vi "test_examples.vi"(9 "expectations":cluster{"label":string, "<JSON>value":string}[](array[cluster]), 10 "controls":cluster{"label":string, "<JSON>value":string}[](array[cluster]), 11 "file":string) -> (0 "error out":errorcluster)   [LabVIEW 2017, in "example_tests.lvlib"]
uses:
  example_tests.lvlib
  de0021a5-3447-4bd8-a116-6765a7690623.vi
  f64fb9af-96c6-48b4-92cc-20c95939fb08.vi
  libssh2/libssh2_init_default.vi
  <vilib>/JDP Science/JSONtext/JSON text to Variant.vi
  <vilib>/JDP Science/JSONtext/Variant to JSON Text.vi
  <vilib>/JDP Science/JSONtext/LVClass Serializer/JSONtext LVClass Serializer.lvclass
  libssh2/libssh2.lvlib
  <vilib>/JDP Science/JSONtext/JSONtext.lvlib
  <vilib>/PNR/Transparent Assertions/Transparent Assertions/Transparent Assertions.lvlib
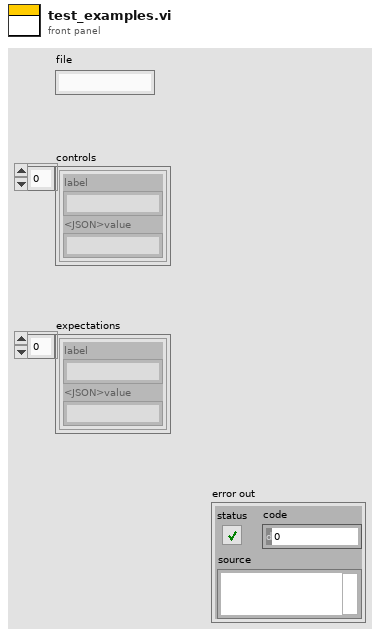
[diagram p1: front panel]
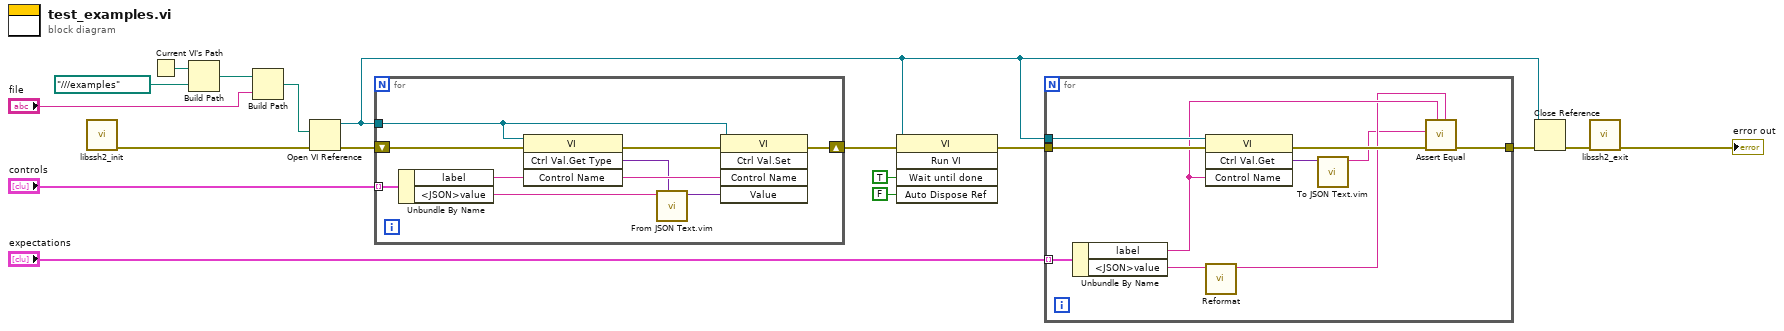
[diagram p0: block diagram]
diagram:
  n1 = call-poly "libssh2_init.vi"() -> ("error out"=w15:errorcluster)  [unwired: 11 in]
  n2 = Current VI's Path() -> (path=w11:path)
  n3 = Build Path(base path=w11, name or relative path=path "../../../examples" ("path")) -> (appended path=w9:path)
  n4 = Build Path(base path=w9, name or relative path="file") -> (appended path=w8:path)
  n5 = Open VI Reference(vi path=w8, error in (no error)=w15) -> (vi reference=w6:refnum<vi>, error out=w13:errorcluster)  [unwired: 4 in]
  n6 = for {
    tunnel: "controls" -> [w26] mode=indexing
    shift-right: [w25] -> w12
    shift-left: w13 -> [w23]
    tunnel: w6 -> [w24]
    n7 = Unbundle By Name(w26) -> ("label"=w22:string, "<JSON>value"=w20:string)
    n8 = invoke on="Invoke Node" class="VI" method="Ctrl Val.Get Type"(reference=w24, error in=w23, "Control Name"=w22) -> (error out=w18:errorcluster, "Ctrl Val.Get Type"=w21:variant)  [unwired: 1 in, 2 out]
    n9 = call "From JSON Text.vim"("Data Type and Default Value"=w21, "JSON"=w20) -> ("Data out"=w19:variant)  [unwired: 8 in, 1 out]
    n10 = invoke on="Invoke Node" class="VI" method="Ctrl Val.Set"(reference=w24, error in=w18, "Control Name"=w22, "Value"=w19) -> (error out=w25:errorcluster)  [unwired: 1 in, 4 out]
  }
  n11 = invoke on="Invoke Node" class="VI" method="Run VI"(reference=w6, error in=w12, "Wait until done"=TRUE ("Wait Until Done"), "Auto Dispose Ref"=FALSE ("Auto Dispose Reference")) -> (error out=w14:errorcluster)  [unwired: 1 in, 4 out]
  n12 = for {
    tunnel: w6 -> [w33]
    tunnel: w14 -> [w36]
    tunnel: [w35] -> w7
    tunnel: "expectations" -> [w34] mode=indexing
    n13 = Unbundle By Name(w34) -> ("label"=w32:string, "<JSON>value"=w31:string)
    n14 = invoke on="Invoke Node" class="VI" method="Ctrl Val.Get"(reference=w33, error in=w36, "Control Name"=w32) -> (error out=w29:errorcluster, "Get Control Value Variant"=w30:variant)  [unwired: 1 in, 2 out]
    n15 = call <vilib>:"Reformat.vi"("JSON"=w31) -> ("<JSON>"=w28:string)  [unwired: 7 in, 3 out]
    n16 = call "To JSON Text.vim"("Anything"=w30) -> ("<JSON>"=w27:string)  [unwired: 9 in, 1 out]
    n17 = call <vilib>:"Assert Equal.vi"("Expected"=w28, "Message (\"\")"=w32, "error in (no error)"=w29, "Actual"=w27) -> ("error out"=w35:errorcluster)  [unwired: 7 in]
  }
  n18 = Close Reference(reference=w6, error in (no error)=w7) -> (error out=w5:errorcluster)
  n19 = call "libssh2_exit.vi"("error in (no error)"=w5) -> ("error out"=→"error out":errorcluster)  [unwired: 10 in]
